vi "Process.vi"(8 "error in":errorcluster, 11 "SynchIO.USB4431":refnum<class "SynchIO.USB4431.lvclass">) -> (0 "error out":errorcluster, 3 "SynchIO.USB4431 out":refnum<class "SynchIO.USB4431.lvclass">)   [LabVIEW 2016, in "SynchIO.USB4431.lvclass"]
doc: "---------------------------------------------------------------\nJKI State Machine Objects™\nhttp://jki.net/state-machine-objects/\nCopyright (C) 2005-2015, JKI <info@jki.net>\nALL RIGHTS RESERVEDJKI State Machine Objects (SMO) 1.0.0.5\nJKI - JKI\nCopyright (c) 2016, JKI"
uses:
  SynchIO.USB4431.lvclass
  C:/Program Files (x86)/National Instruments/LabVIEW 2016/vi.lib/JKI/JKI SMO/SMO/SMO.lvclass
  <vilib>/JKI/JKI SMO/SMO/Typedefs/Parent Call--Enum.ctl
  SynchIO/SynchIO.lvclass
  <vilib>/JKI/JKI SMO/SMO/SMO.lvclass
panel:
  in  "Start":bool
  in  "stop":bool
  in  "Tab Control":T1(tab)=enum."AO Config"
  in  "AI Configuration":T2(array[cluster])=[{"AI.Coupling"=enum."DC", "AI.Max"=10.0, "AI.Min"=-10.0, "Input physical channels"="Dev1/ai0:3"}]
  in  "AO Configuration":T3(array[cluster])=[{"Output physical channels"="Dev1/ao0", "AO. Max"=3.5, "AO.Min"=-3.5}]
  in  "sampling info":cluster{"Fs":dbl, "#s":dbl}={"Fs"=102388.0, "#s"=7876.0}
  in  "AI Buffer Size (S)":i32=100
  in  "Channels: AO":T4={"AO amp (V)"=[1.0, 0.0, 0.0, 0.0, 0.0, 0.0, 0.0, 0.0], "AO DC (V)"=[0.0, 0.0, 0.0, 0.0, 0.0, 0.0, 0.0, 0.0], "AO f (Hz)"=[17.0, 13.0, 13.0, 13.0, 13.0, 13.0, 13.0, 13.0], "AO phi (deg)"=[0.0, 0.0, 0.0, 0.0, 0.0, 0.0, 0.0, 0.0], "function"=[enum."Sine Wave", enum."Sine Wave", enum."Sine Wave", enum."Sine Wave", enum."Sine Wave", enum."Sine Wave", enum."Sine Wave", enum."Sine Wave"]}
  in  "AO":T4={"AO amp (V)"=[1.0, 0.0, 0.0, 0.0, 0.0, 0.0, 0.0, 0.0], "AO DC (V)"=[0.0, 0.0, 0.0, 0.0, 0.0, 0.0, 0.0, 0.0], "AO f (Hz)"=[13.0, 13.0, 13.0, 13.0, 13.0, 13.0, 13.0, 13.0], "AO phi (deg)"=[0.0, 0.0, 0.0, 0.0, 0.0, 0.0, 0.0, 0.0], "function"=[enum."Sine Wave", enum."Sine Wave", enum."Sine Wave", enum."Sine Wave", enum."Sine Wave", enum."Sine Wave", enum."Sine Wave", enum."Sine Wave"]} {"AO DC (V)" format="%#_6p"; "AO amp (V)" format="%#_6p"}
  out "Signals Graph":waveform(dbl)[](graph)=[{"t0"=timestamp(3565974471.4961195 s since 1904-01-01), "dt"=1.0, "Y"=array[6023 elements], "attributes"=variant("NI_ChannelName"=variant(string "Dev2/ai0"), "NI_UnitDescription"=variant(string "Volts"))}, {"t0"=timestamp(3565974471.4961195 s since 1904-01-01), "dt"=1.0, "Y"=array[6023 elements], "attributes"=variant("NI_ChannelName"=variant(string "Dev2/ai1"), "NI_UnitDescription"=variant(string "Volts"))}, {"t0"=timestamp(3565974471.4961195 s since 1904-01-01), "dt"=1.0, "Y"=array[6023 elements], "attributes"=variant("NI_ChannelName"=variant(string "Dev2/ai2"), "NI_UnitDescription"=variant(string "Volts"))}, {"t0"=timestamp(3565974471.4961195 s since 1904-01-01), "dt"=1.0, "Y"=array[6023 elements], "attributes"=variant("NI_ChannelName"=variant(string "Dev2/ai3"), "NI_UnitDescription"=variant(string "Volts"))}, {"t0"=timestamp(3565974471.554943 s since 1904-01-01), "dt"=1.0, "Y"=array[6023 elements], "attributes"=variant("NI_ChannelName"=variant(string "Dev2/ai0"), "NI_UnitDescription"=variant(string "Volts"))}, {"t0"=timestamp(3565974471.554943 s since 1904-01-01), "dt"=1.0, "Y"=array[6023 elements], "attributes"=variant("NI_ChannelName"=variant(string "Dev2/ai1"), "NI_UnitDescription"=variant(string "Volts"))}]
  out "Signals Graph 2":waveform(dbl)[](graph)=[{"t0"=timestamp(3565974471.4961195 s since 1904-01-01), "dt"=1.0, "Y"=array[6023 elements], "attributes"=variant("NI_ChannelName"=variant(string "Dev2/ai0"), "NI_UnitDescription"=variant(string "Volts"))}, {"t0"=timestamp(3565974471.4961195 s since 1904-01-01), "dt"=1.0, "Y"=array[6023 elements], "attributes"=variant("NI_ChannelName"=variant(string "Dev2/ai1"), "NI_UnitDescription"=variant(string "Volts"))}, {"t0"=timestamp(3565974471.4961195 s since 1904-01-01), "dt"=1.0, "Y"=array[6023 elements], "attributes"=variant("NI_ChannelName"=variant(string "Dev2/ai2"), "NI_UnitDescription"=variant(string "Volts"))}, {"t0"=timestamp(3565974471.4961195 s since 1904-01-01), "dt"=1.0, "Y"=array[6023 elements], "attributes"=variant("NI_ChannelName"=variant(string "Dev2/ai3"), "NI_UnitDescription"=variant(string "Volts"))}, {"t0"=timestamp(3565974471.554943 s since 1904-01-01), "dt"=1.0, "Y"=array[6023 elements], "attributes"=variant("NI_ChannelName"=variant(string "Dev2/ai0"), "NI_UnitDescription"=variant(string "Volts"))}, {"t0"=timestamp(3565974471.554943 s since 1904-01-01), "dt"=1.0, "Y"=array[6023 elements], "attributes"=variant("NI_ChannelName"=variant(string "Dev2/ai1"), "NI_UnitDescription"=variant(string "Volts"))}]
  out "Current State":string="Exit"
  out "State History":string
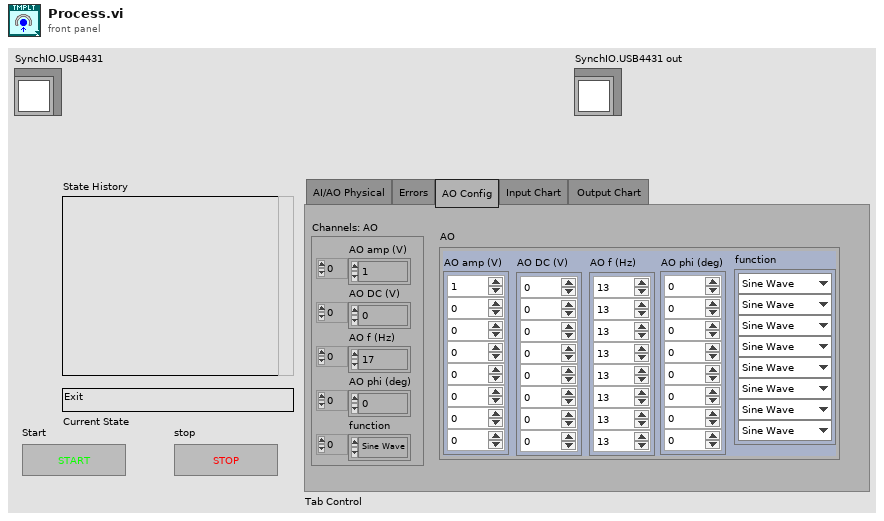
[diagram p1: front panel]
types:
  T1 = enum32{"AI/AO Physical", "Errors", "AO Config", "Input Chart", "Output Chart "}
  T2 = cluster{"AI.Coupling":enum16{"AC", "DC", "GND"}, "AI.Max":dbl, "AI.Min":dbl, "Input physical channels":tag}[]
  T3 = cluster{"Output physical channels":tag, "AO. Max":dbl, "AO.Min":dbl}[]
  T4 = cluster{"AO amp (V)":dbl[], "AO DC (V)":dbl[], "AO f (Hz)":dbl[], "AO phi (deg)":dbl[], "function":enum16{"Sine Wave", "Triangle Wave", "Square Wave", "Sawtooth Wave"}[]}
  T5 = typedef "SMO.lvclass/Parent Call--Enum.ctl" = enum16{"Allows parent to run", "Does not request parent to run"}
  T6 = enum32{"invalid app kind", "Development System", "Run Time System", "Student Edition", "Embedded LabVIEW", "Evaluation", "Custom"}
  T7 = enum32{"Invalid", "Standard", "Closed", "Hidden", "Minimized", "Maximized"}
  T8 = cluster{"Core":cluster{"Current VI Reference":refnum<vi>, "Close Panel on Exit?":bool, "error":errorcluster}, "Self Reference":refnum<class "SynchIO.USB4431.lvclass">, "Your string data":string, "AI Buffer Size (S)":i32, "AI Configuration":cluster{"AI.Coupling":enum16{"AC", "DC", "GND"}, "AI.Max":dbl, "AI.Min":dbl, "Input physical channels":tag}[], "AO Configuration":cluster{"Output physical channels":tag, "AO. Max":dbl, "AO.Min":dbl}[], "Channels: AO":cluster{"AO amp (V)":dbl[], "AO DC (V)":dbl[], "AO f (Hz)":dbl[], "AO phi (deg)":dbl[], "function":enum16{"Sine Wave", "Triangle Wave", "Square Wave", "Sawtooth Wave"}[]}, "sampling info":cluster{"Fs":dbl, "#s":dbl}, "AI task":refnum<k21>[], "AO Task":refnum<k21>[], "AI Data":waveform(dbl)[], "AO Data":waveform(dbl)[], "AO":cluster{"AO amp (V)":dbl[], "AO DC (V)":dbl[], "AO f (Hz)":dbl[], "AO phi (deg)":dbl[], "function":enum16{"Sine Wave", "Triangle Wave", "Square Wave", "Sawtooth Wave"}[]}, "Iteration":i32}
  T9 = cluster{"Current VI Reference":refnum<vi>, "Close Panel on Exit?":bool, "error":errorcluster}
  T10 = typedef "SMO.lvclass/Protected Events.ctl" = cluster{"StopProcesses":refnum<user-event>, "AbortProcesses":refnum<user-event>, "Config Changed":refnum<user-event>, "Dependency":refnum<user-event>}
  T11 = typedef "SynchIO.USB4431.lvclass/ProtectedEvents--Cluster.ctl" = cluster{"API_Template":refnum<user-event>}
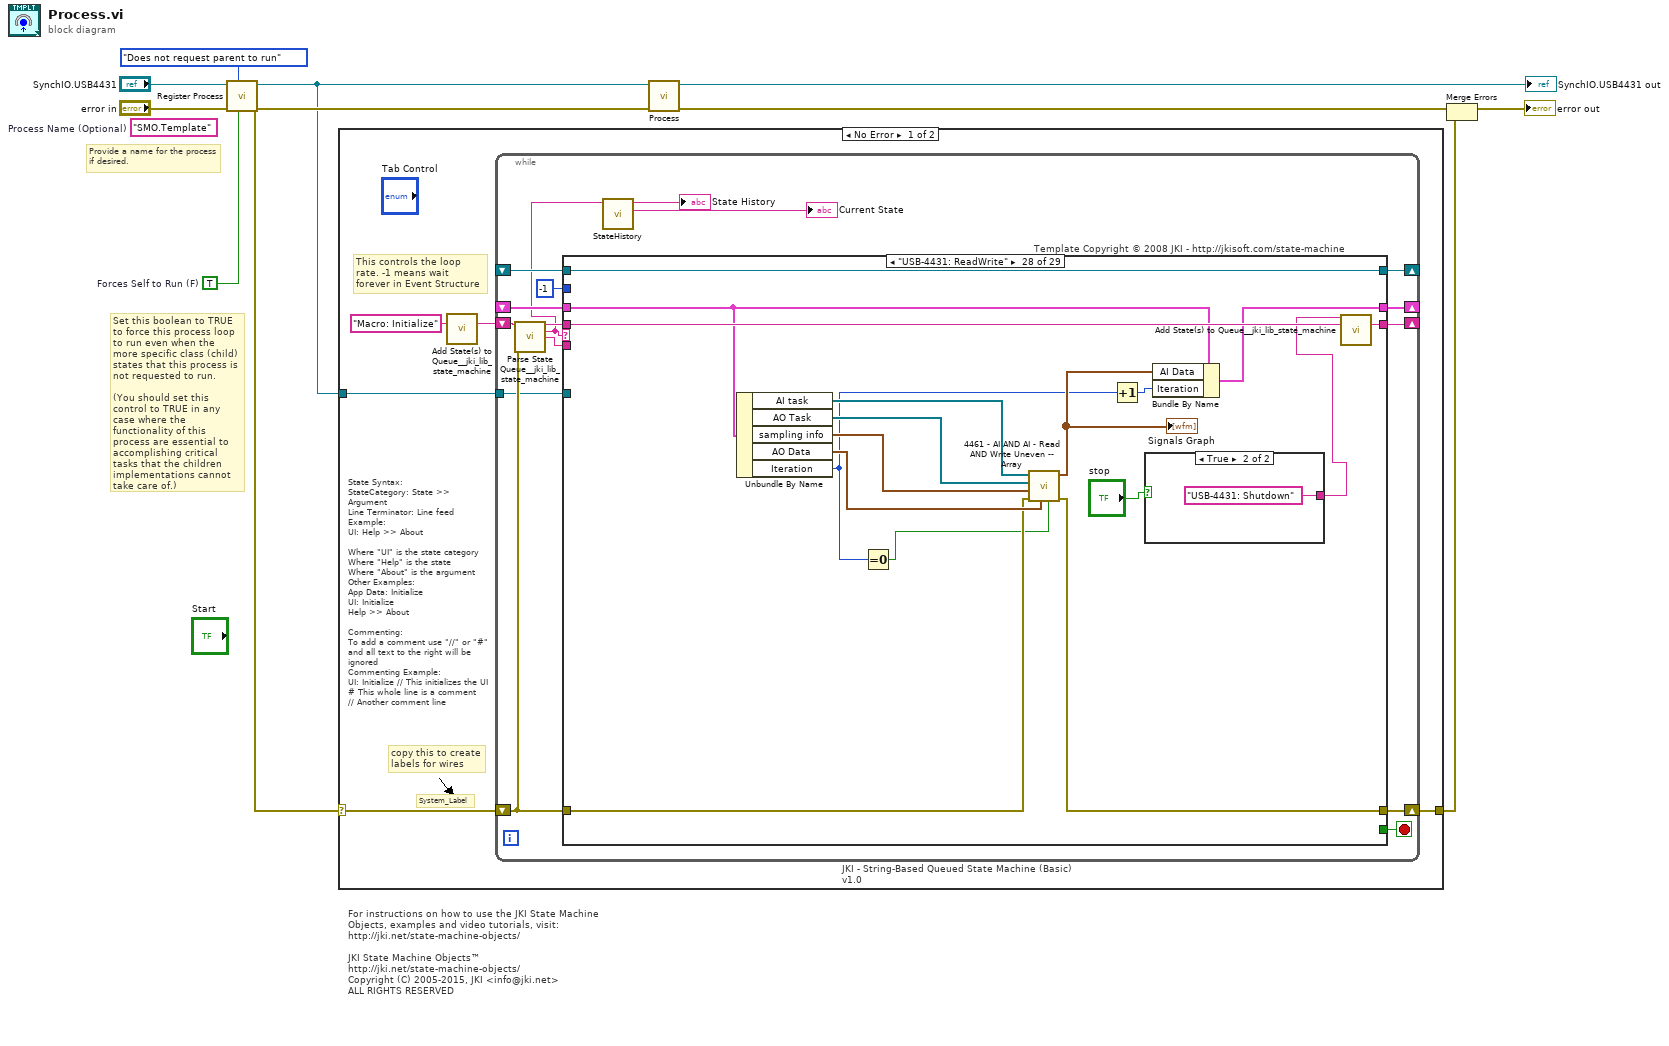
[diagram p0: block diagram]
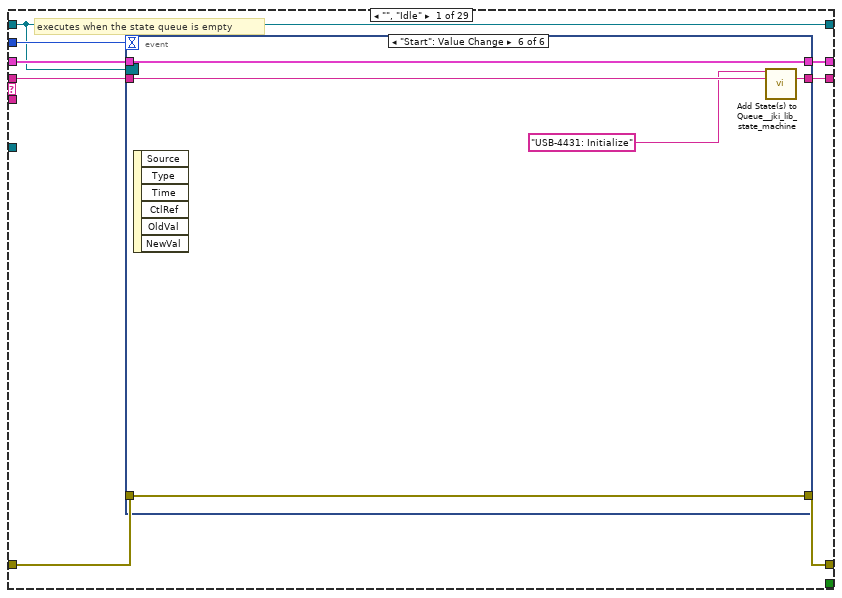
[diagram p2: hidden frame]
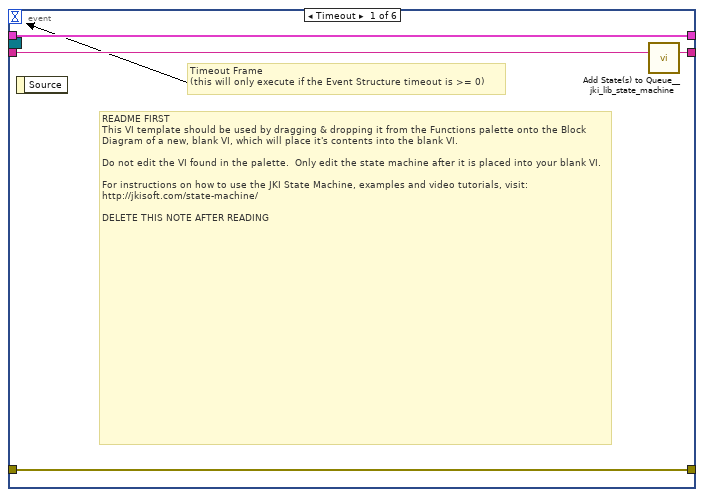
[diagram p3: hidden frame]
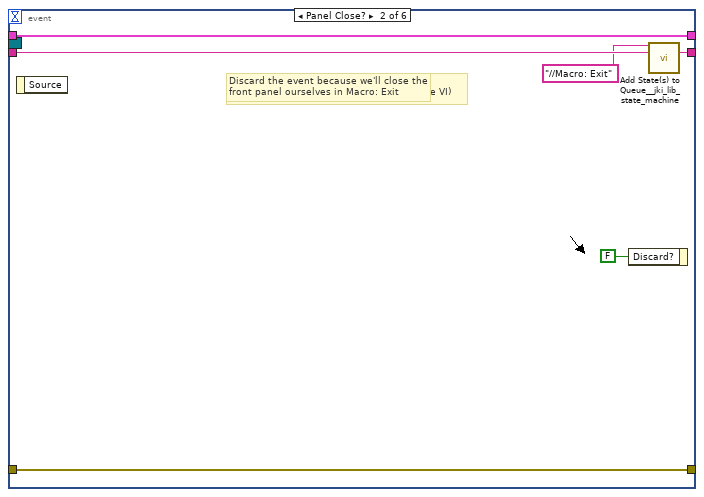
[diagram p4: hidden frame]
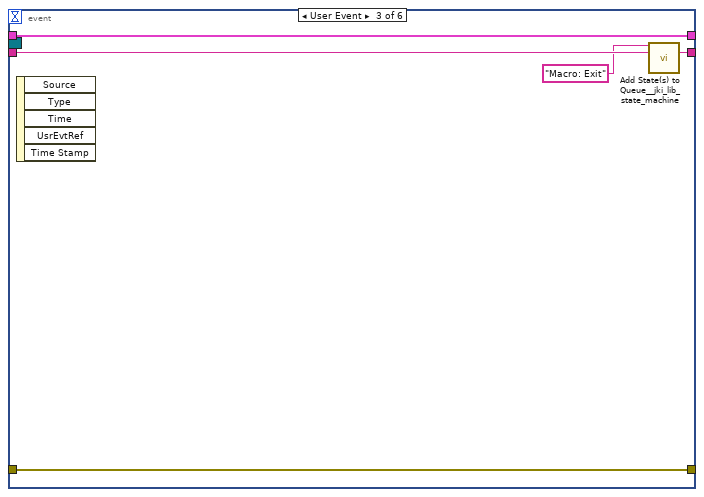
[diagram p5: hidden frame]
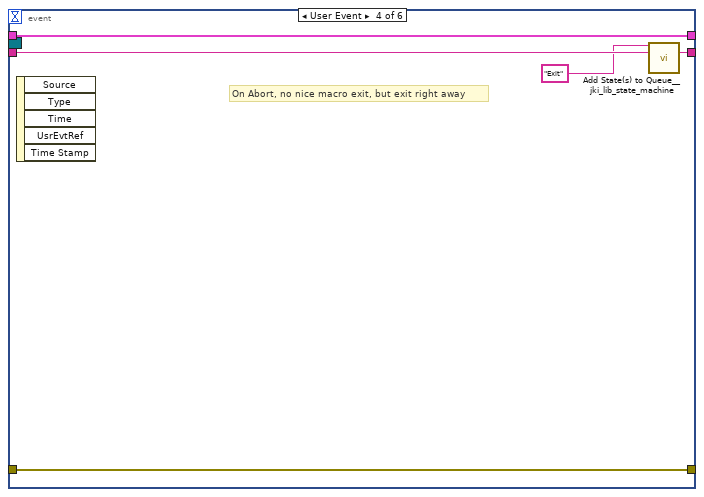
[diagram p6: hidden frame]
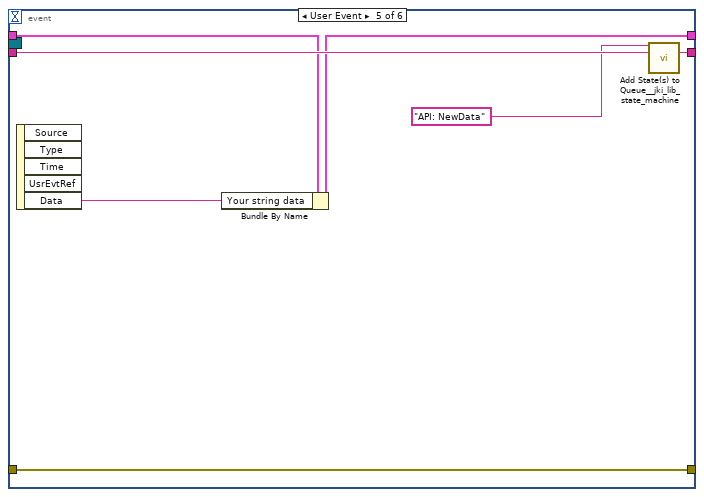
[diagram p7: hidden frame]
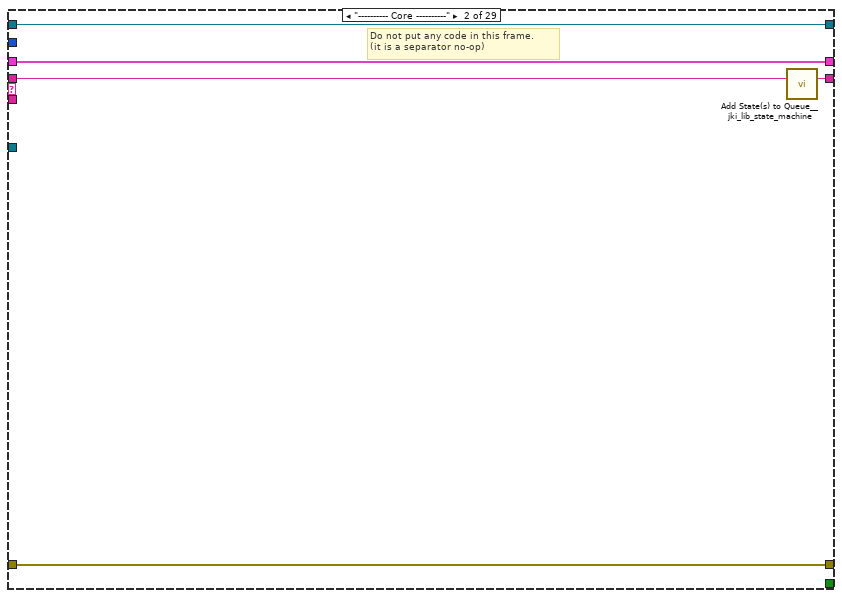
[diagram p8: hidden frame]
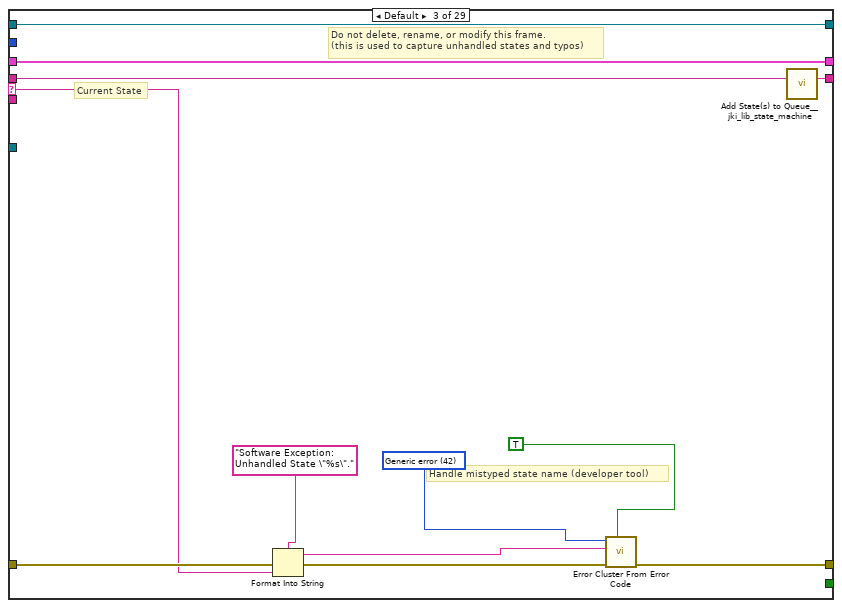
[diagram p9: hidden frame]
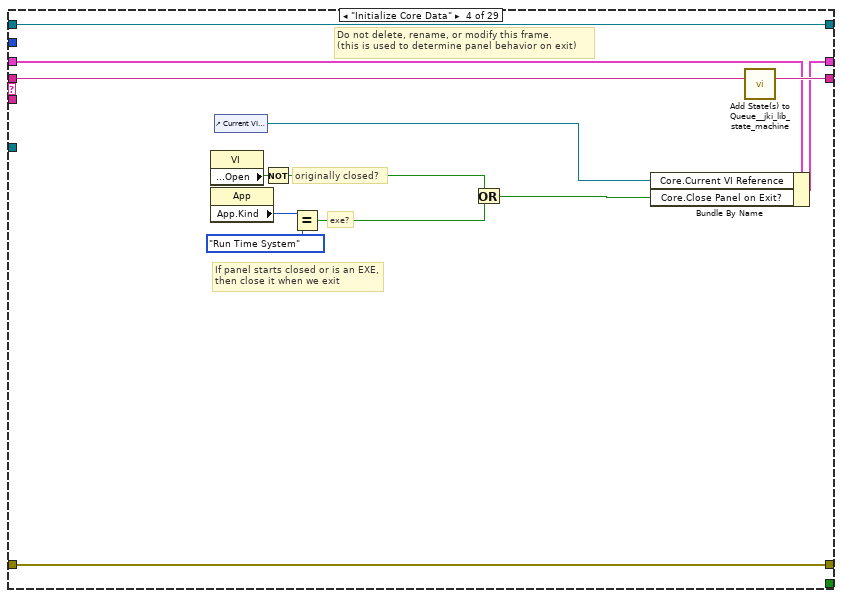
[diagram p10: hidden frame]
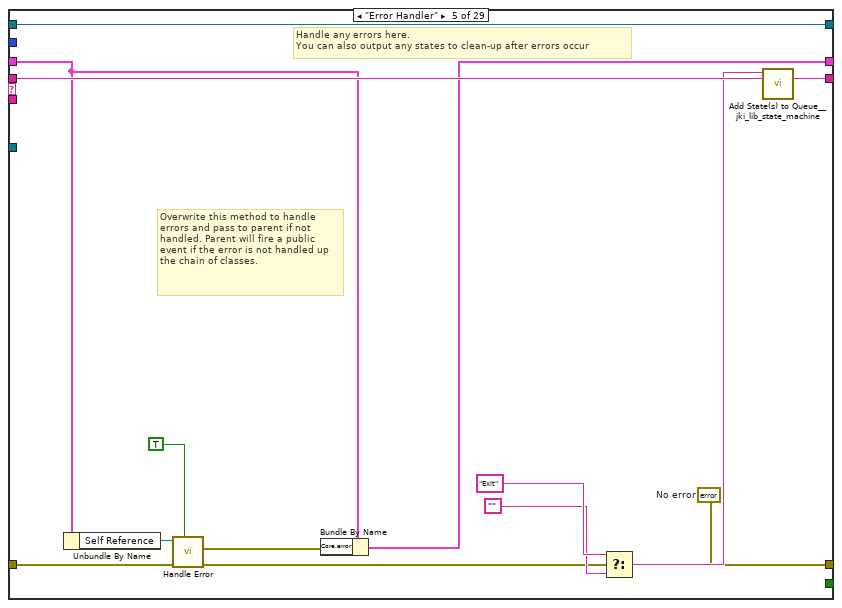
[diagram p11: hidden frame]
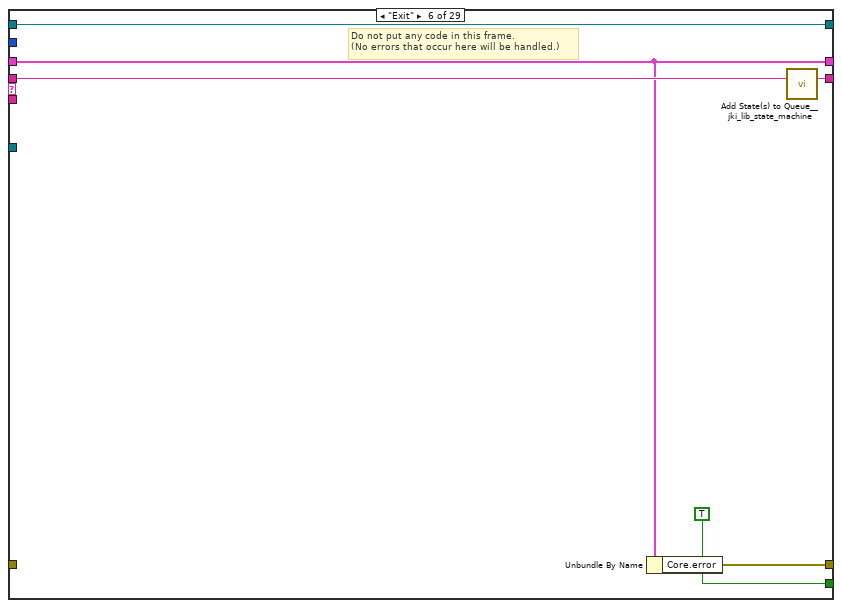
[diagram p12: hidden frame]
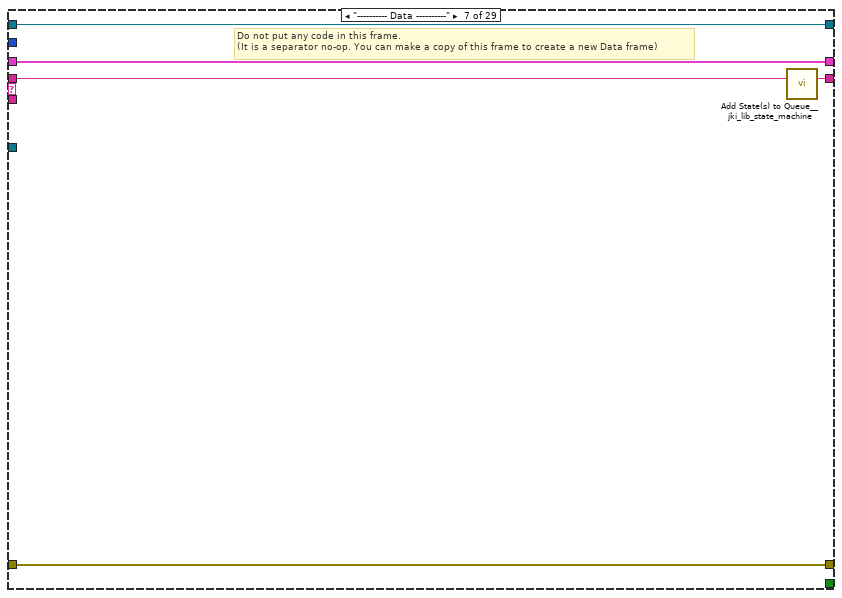
[diagram p13: hidden frame]
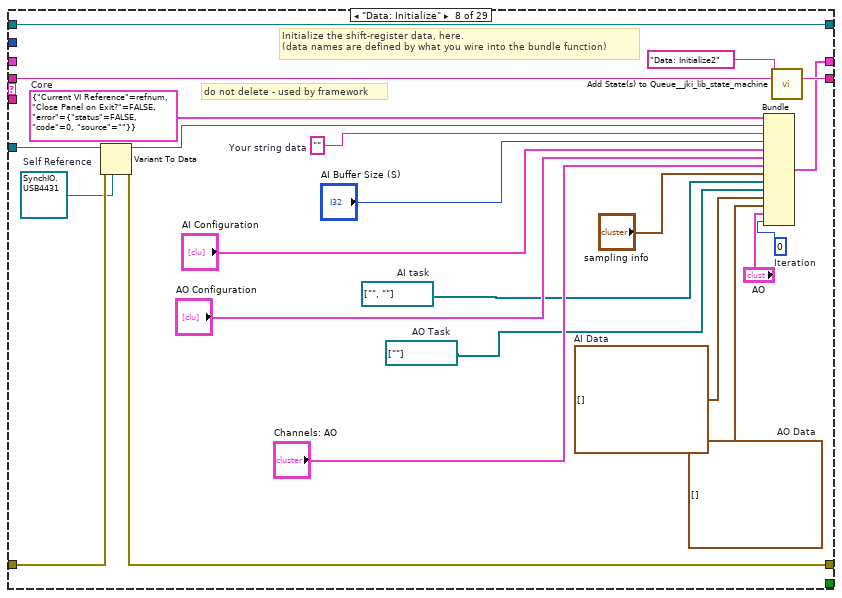
[diagram p14: hidden frame]
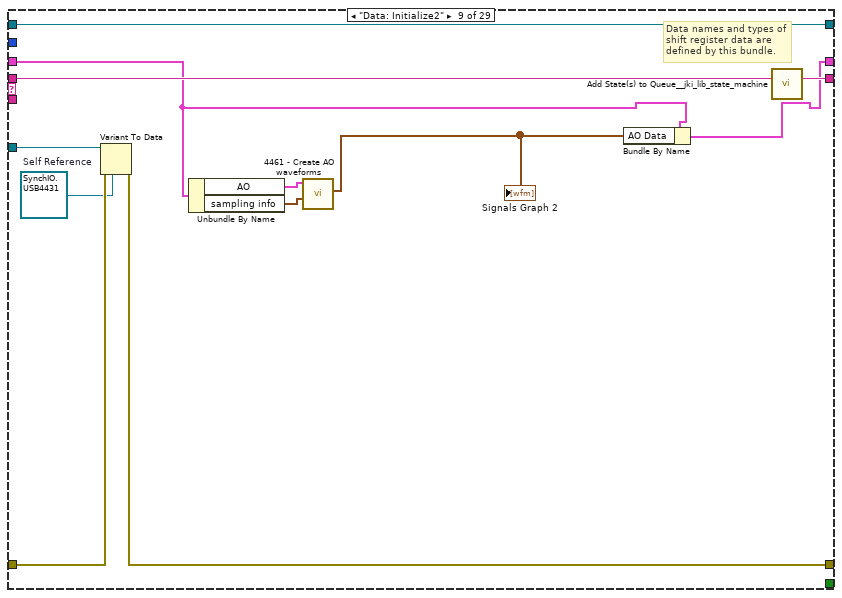
[diagram p15: hidden frame]
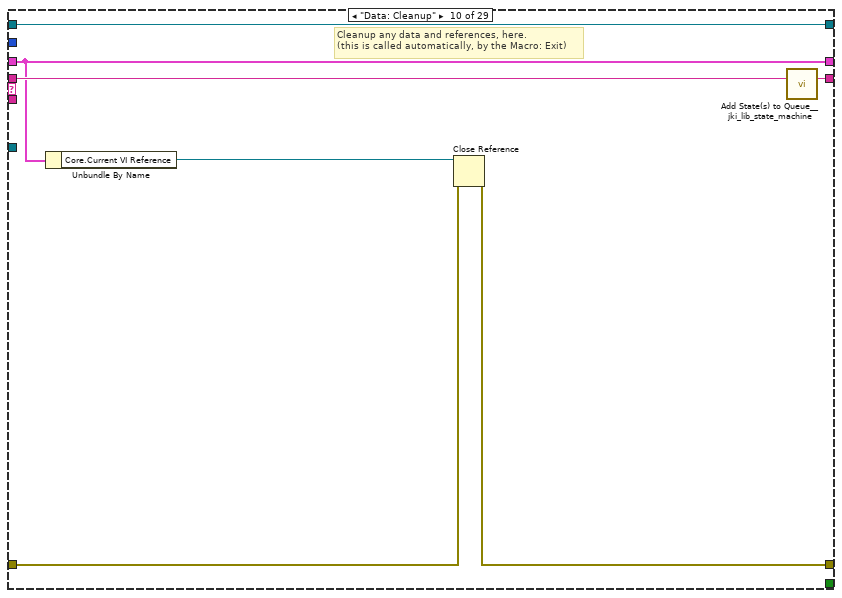
[diagram p16: hidden frame]
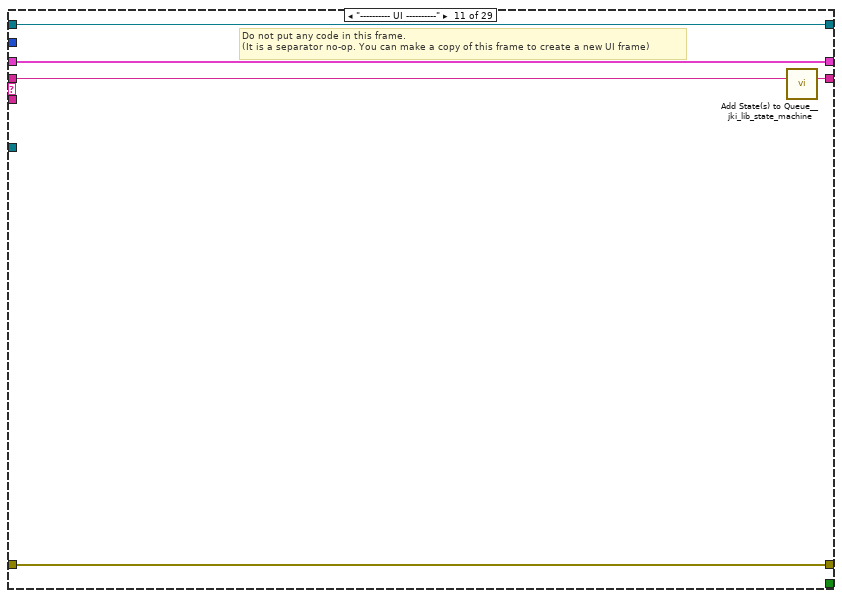
[diagram p17: hidden frame]
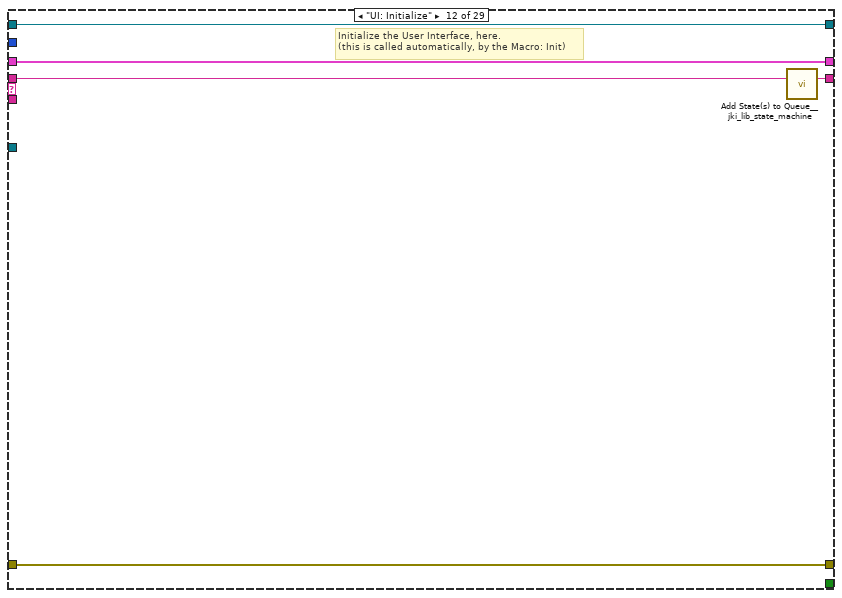
[diagram p18: hidden frame]
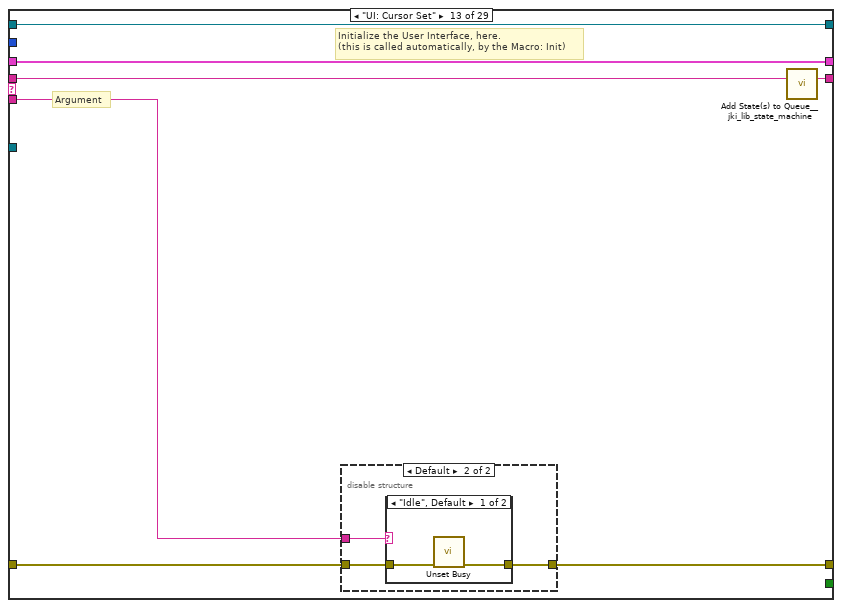
[diagram p19: hidden frame]
diagram:
  w1 = TRUE  # Forces Self to Run (F)
  (unwired) "SMO.Template"  # Process Name (Optional)
  # "Provide a name for the process\nif desired."
  # "Set this boolean to TRUE to force this process loop to run even when the more specific class (child) states that this process is not requested to run.\n\n(You should set this control to TRUE in any case where the functionality of this process are essential to accomplishing critical tasks that the children implementations cannot take care of.)"
  # "For instructions on how to use the JKI State Machine Objects, examples and video tutorials, visit:\nhttp://jki.net/state-machine-objects/\n\nJKI State Machine Objects™\nhttp://jki.net/state-machine-objects/\nCopyright (C) 2005-2015, JKI <info@jki.net>\nALL RIGHTS RESERVED"
  n1 = call <vilib>:"Register Process.vi"("Forces Self to Run (F)"=w1, "Parent Call"=Parent_Call--Enum."Does not request parent to run", "error in (no error)"="error in", "SMO"="SynchIO.USB4431") -> ("error out"=w7:errorcluster, "SMO out"=w6:refnum<class "SynchIO.USB4431.lvclass">)  [unwired: 6 in]
  n2 = case shown="No Error" w7 {
    selector: w7 -> [w12 w378]
    tunnel: w6 -> [w13 _]
    tunnel: [w11 w378] -> w3
    frame No Error {
      # "State Syntax:\nStateCategory: State >> Argument\nLine Terminator: Line feed\nExample:\nUI: Help >> About\n\nWhere \"UI\" is the state category\nWhere \"Help\" is the state\nWhere \"About\" is the argument\nOther Examples:\nApp Data: Initialize\nUI: Initialize\nHelp >> About\n\nCommenting:\nTo add a comment use \"//\" or \"#\" and all text to the right will be ignored\nCommenting Example:\nUI: Initialize // This initializes the UI\n# This whole line is a comment\n// Another comment line"
      # "copy this to create labels for wires"
      # "This controls the loop rate. -1 means wait forever in Event Structure"
      # "System_Label"
      n3 = call <vilib>:"Add State(s) to Queue__jki_lib_state_machine.vi"("State(s) in (\"\")"="Macro: Initialize") -> ("States Out"=w15:string)  [unwired: 14 in]
      n4 = while "JKI - String-Based Queued State Machine (Basic) v1.0" {
        shift-right: [w26] -> _
        shift-left: _ -> [w25]
        shift-right: [w29] -> w11
        shift-left: w12 -> [w23]
        shift-right: [w28] -> _
        shift-left: w15 -> [w30]
        tunnel: w13 -> [w22]
        shift-right: [w21] -> _
        shift-left: _ -> [w20]
        stop <- w27 stop-if-true
        # "Template Copyright © 2008 JKI - http://jkisoft.com/state-machine"
        n5 = call <vilib>:"Parse State Queue__jki_lib_state_machine.vi"("State Queue"=w30, "Error In (no error)"=w23) -> ("Remaining States"=w17:string, "Current State"=w16:string, "Arguments"=w31:string)  [unwired: 11 in]
        n6 = case shown="\"USB-4431: ReadWrite\"" w16 {
          selector: w16 -> [_ _ w78 _ _ _ _ _ _ _ _ _ _ _ _ _ _ _ _ _ _ _ _ _ _ _ _ _ _]
          tunnel: w17 -> [w39 w76 w82 w101 w115 w121 w126 w149 w161 w168 w173 w178 w185 w201 w233 w242 w256 w261 w272 w277 w290 w296 w301 w309 w314 w319 w335 w352 w364]
          tunnel: w31 -> [_ _ _ _ _ _ _ _ _ _ _ _ w179 w195 _ _ _ _ _ _ _ _ _ _ _ _ _ _ _]
          tunnel: w25 -> [w37 w73 w80 w92 w104 w117 w123 _ w152 w163 w170 w176 w183 w197 w230 w238 w247 w258 w269 w274 w288 w294 w299 w306 w311 w317 w328 w349 w359]
          tunnel: [w36 w74 w84 w98 w106 w116 w124 w144 w158 w164 w171 w175 w180 w198 w231 w240 w254 w259 w263 w275 w278 w292 w297 w303 w310 w315 w324 w344 w361] -> w29
          tunnel: w23 -> [w35 w74 w83 w98 w111 _ w124 w145 w159 w165 w171 w175 w181 w199 w231 w240 w254 w259 w264 w275 w282 w292 w297 w304 w310 w315 w325 w339 w360]
          tunnel: [w38 w75 w81 w100 w114 w120 w125 w148 w160 w167 w172 w177 w184 w200 w232 w241 w255 w260 w271 w276 w289 w295 w300 w308 w313 w318 w334 w351 w363] -> w28
          tunnel: [_ _ _ _ _ TRUE _ _ _ _ _ _ _ _ _ _ _ _ _ _ _ _ _ _ _ _ _ _ _] -> w27
          tunnel: [w34 w73 w80 w99 w103 w117 w123 w147 w151 w163 w170 w176 w183 w197 w230 w238 w247 w258 w269 w274 w288 w294 w299 w306 w311 w317 w327 w348 w359] -> w26
          tunnel: -1 ("Timeout") -> [w33 _ _ _ _ _ _ _ _ _ _ _ _ _ _ _ _ _ _ _ _ _ _ _ _ _ _ _ _]
          tunnel: w22 -> [_ _ _ _ _ _ _ w142 w156 _ _ _ _ _ _ _ _ _ _ _ _ _ _ _ _ _ _ _ _]
          tunnel: [w32 w72 w77 w89 w113 w118 w122 w140 w155 w162 w169 w174 w182 w194 w229 w239 w248 w257 w270 w273 w287 w293 w298 w307 w312 w316 w333 w350 w362] -> w21
          tunnel: w20 -> [w32 w72 w77 w89 w113 w118 w122 w140 w155 w162 w169 w174 w182 w194 w229 w239 w248 w257 w270 w273 _ w293 w298 w307 w312 w316 w333 w350 w362]
          frame "", "Idle" {
            # "executes when the state queue is empty"
            n7 = event shown="[5] \"Start\": Value Change" {
              selector: w32 -> [_ _ _ _ _ _]
              dyn-events: _ -> [_ _ _ _ _ _]
              timeout: w33 -> [_ _ _ _ _ _]
              tunnel: w39 -> [w43 w49 w54 w59 w66 w71]
              tunnel: [w42 w48 w53 w58 w65 w70] -> w38
              tunnel: w37 -> [w40 w46 w51 w56 w63 w67]
              tunnel: [w41 w47 w52 w57 w64 w69] -> w36
              tunnel: w35 -> [w41 w47 w52 w57 w64 w69]
              tunnel: [w40 w46 w51 w56 w62 w67] -> w34
              event Timeout {
                # "README FIRST\nThis VI template should be used by dragging & dropping it from the Functions palette onto the Block Diagram of a new, blank VI, which will place it's contents into the blank VI.\n\nDo not edit the VI found in the palette.  Only edit the state machine after it is placed into your blank VI.\n\nFor instructions on how to use the JKI State Machine, examples and video tutorials, visit:\nhttp://jkisoft.com/state-machine/\n\nDELETE THIS NOTE AFTER READING"
                # "Timeout Frame\n(this will only execute if the Event Structure timeout is >= 0)"
                n8 = event-data() -> ()  [unwired: 1 in, 1 out]
                n9 = call <vilib>:"Add State(s) to Queue__jki_lib_state_machine.vi"("State(s) in (\"\")"=w43) -> ("States Out"=w42:string)  [unwired: 14 in]
              }
              event Panel Close? {
                # "Discard the event because we'll close the front panel ourselves in Macro: Exit"
                # "Close Panel button (pressed) Event\n(this executes Macro: Exit to terminate the VI)"
                n10 = event-data() -> ()  [unwired: 1 in, 1 out]
                n11 = event-data("Discard?"=FALSE) -> ()  [unwired: 1 in, 1 out]
                n12 = call <vilib>:"Add State(s) to Queue__jki_lib_state_machine.vi"("State(s) in Front (\"\")"="//Macro: Exit", "State(s) in (\"\")"=w49) -> ("States Out"=w48:string)  [unwired: 13 in]
              }
              event User Event {
                n13 = event-data() -> ()  [unwired: 1 in, 5 out]
                n14 = call <vilib>:"Add State(s) to Queue__jki_lib_state_machine.vi"("State(s) in Front (\"\")"="Macro: Exit", "State(s) in (\"\")"=w54) -> ("States Out"=w53:string)  [unwired: 13 in]
              }
              event User Event {
                # "On Abort, no nice macro exit, but exit right away"
                n15 = event-data() -> ()  [unwired: 1 in, 5 out]
                n16 = call <vilib>:"Add State(s) to Queue__jki_lib_state_machine.vi"("State(s) in Front (\"\")"="Exit", "State(s) in (\"\")"=w59) -> ("States Out"=w58:string)  [unwired: 13 in]
              }
              event User Event {
                n17 = event-data() -> ("Data"=w60:string)  [unwired: 1 in, 4 out]
                n18 = Bundle By Name(cluster=w63, "Your string data"=w60) -> (w62:T8)
                n19 = call <vilib>:"Add State(s) to Queue__jki_lib_state_machine.vi"("State(s) in Front (\"\")"="API: NewData", "State(s) in (\"\")"=w66) -> ("States Out"=w65:string)  [unwired: 13 in]
              }
              event "Start": Value Change {
                n20 = event-data() -> ()  [unwired: 1 in, 6 out]
                n21 = call <vilib>:"Add State(s) to Queue__jki_lib_state_machine.vi"("State(s) in Front (\"\")"="USB-4431: Initialize", "State(s) in (\"\")"=w71) -> ("States Out"=w70:string)  [unwired: 13 in]
              }
            }
          }
          frame "---------- Core ----------" {
            # "Do not put any code in this frame.\n(it is a separator no-op)"
            n22 = call <vilib>:"Add State(s) to Queue__jki_lib_state_machine.vi"("State(s) in (\"\")"=w76) -> ("States Out"=w75:string)  [unwired: 14 in]
          }
          frame Default {
            w87 = 42 items=["No error", "Argument error", "Memory is full", "Out of zone", "End of file", "File already open", "Generic file I/O error", "File not found", "File permission error", "Disk is full", "Duplicate path", "Too many files open", "System feature not enabled", "Resource file not found", "Cannot add resource", "Resource not found", "Image not found", "Image memory error", "Pen does not exist", "Config type invalid", "Config token not found", "Config parse error", "Config memory error", "Bad external code format", "Bad external code offset", "External code not present", "Null window", "Destroy window error", "Null menu", "Print aborted", "Bad print record", "Print driver error", "Windows error during printing", "Memory error during printing", "Print dialog error", "Generic print error", "Invalid device refnum", "Device not found", "Device parameter error", "Device unit error", "Cannot open device", "Device call aborted", "Generic error", "Cancelled by user", "Object ID too low", "Object ID too high", "Object not in heap", "Unknown heap", "Unknown object (invalid DefProc)", "Unknown object (DefProc not in table)", "Message out of range", "Invalid (null) method", "Unknown message", "Manager call not supported", "Bad address", "Network operation in progress", "Network operation timed out", "Connection is busy", "Network attribute not supported", "Network error", "Address in use", "System out of memory", "Connection aborted", "Connection refused", "Not connected", "Already connected", "Connection closed", "Initialization error (interapplication manager)", "Bad occurrence", "Wait on unbound occurrence handler", "Occurrence queue overflow", "Datalog type conflict", "Unused", "Unrecognized type (interapplication manager)", "Memory corrupt", "Failed to make temporary DLL", "Old CIN version", "Drag socket not found", "Failed to load drop-object", "Failed to register OLE object", "Failed to release OLE object", "Format specifier type mismatch", "Unknown format specifier", "Too few format specifiers", "Too many format specifiers", "Scan failed", "Newer CIN version", "Error converting to variant", "Runtime menu error", "Password tampered", "Variant attribute not found", "Incompatible variant data type", "Event data is not available", "Event Store is not present", "Occurrence is not found", "Event Queue is not created", "Event info is not available", "Refnum passed is NULL", "Error retrieving Class GUID", "Error retrieving CoClass GUID", "Error retrieving TypeLib GUID.", "Bad built application magic bytes.", "Specific driver is different from the specific driver associated with the Logical Name.", "There is no session opened to the class driver.", "Max Error", "MAX - Error with config objects", "MAX - Error loading configuration", "MAX - Group not supported"]
            # "Current State"
            # "Do not delete, rename, or modify this frame.\n(this is used to capture unhandled states and typos)"
            # "Handle mistyped state name (developer tool)"
            n23 = Format Into String(format string="Software Exception: Unhandled State \"%s\"." ("message"), error in=w83, w78) -> (resulting string=w86:string, error out=w85:errorcluster)  [unwired: 1 in]
            n24 = call <vilib>:"Error Cluster From Error Code.vi"("show call chain? (False)"=TRUE, "error in (no error)"=w85, "error message (\"\")"=w86, "error code (0)"=w87) -> ("error out"=w84:errorcluster)  [unwired: 5 in]
            n25 = call <vilib>:"Add State(s) to Queue__jki_lib_state_machine.vi"("State(s) in (\"\")"=w82) -> ("States Out"=w81:string)  [unwired: 14 in]
          }
          frame "Initialize Core Data" {
            # "Do not delete, rename, or modify this frame.\n(this is used to determine panel behavior on exit)"
            # "originally closed?"
            # "exe?"
            # "If panel starts closed or is an EXE, then close it when we exit"
            n26 = property class="VI"() -> ("Front Panel.Open"=w97:bool)  [unwired: 2 in, 2 out]
            n27 = property class="App"() -> ("App.Kind"=w96:T6)  [unwired: 2 in, 2 out]
            n28 = control-ref of="Current VI Reference"() -> (w90:refnum<vi>)
            n29 = Not(x=w97) -> (.not. x?=w94:bool)
            n30 = Equal?(x=w96, y=T6."Run Time System" ("Application:Kind")) -> (x = y?=w93:bool)
            n31 = Or(x=w94, y=w93) -> (x .or. y?=w91:bool)
            n32 = Bundle By Name(cluster=w92, "Core.Current VI Reference"=w90, "Core.Close Panel on Exit?"=w91) -> (w99:T8)
            n33 = call <vilib>:"Add State(s) to Queue__jki_lib_state_machine.vi"("State(s) in (\"\")"=w101) -> ("States Out"=w100:string)  [unwired: 14 in]
          }
          frame "Error Handler" {
            w106 = errorcluster {"status"=FALSE, "code"=0, "source"=""}  # No error
            # "Overwrite this method to handle errors and pass to parent if not handled. Parent will fire a public event if the error is not handled up the chain of classes."
            # "Handle any errors here.\nYou can also output any states to clean-up after errors occur"
            n34 = Unbundle By Name(w104) -> ("Self Reference"=w112:refnum<class "SynchIO.USB4431.lvclass">)
            n35 = call-dynamic "Handle Error.vi"("Stop on Unhandled Error (T)"=TRUE, "error in"=w111, "SMO"=w112) -> ("handling error"=w107:errorcluster, "Unhandled error"=w105:errorcluster)  [unwired: 6 in, 1 out]
            n36 = Bundle By Name(cluster=w104, "Core.error"=w105) -> (w103:T8)
            n37 = Select(t="Exit", s=w107, f="") -> (s? t:f=w108:string)
            n38 = call <vilib>:"Add State(s) to Queue__jki_lib_state_machine.vi"("State(s) in Front (\"\")"=w108, "State(s) in (\"\")"=w115) -> ("States Out"=w114:string)  [unwired: 13 in]
          }
          frame "Exit" {
            # "Do not put any code in this frame.\n(No errors that occur here will be handled.)"
            n39 = Unbundle By Name(w117) -> ("Core.error"=w116:errorcluster)
            n40 = call <vilib>:"Add State(s) to Queue__jki_lib_state_machine.vi"("State(s) in (\"\")"=w121) -> ("States Out"=w120:string)  [unwired: 14 in]
          }
          frame "---------- Data ----------" {
            # "Do not put any code in this frame.\n(It is a separator no-op. You can make a copy of this frame to create a new Data frame)"
            n41 = call <vilib>:"Add State(s) to Queue__jki_lib_state_machine.vi"("State(s) in (\"\")"=w126) -> ("States Out"=w125:string)  [unwired: 14 in]
          }
          frame "Data: Initialize" {
            w127 = 0  # Iteration
            w129 = waveform(dbl)[] []  # AO Data
            w130 = refnum<k21>[] [""]  # AO Task
            w131 = refnum<k21>[] ["", ""]  # AI task
            w135 = waveform(dbl)[] []  # AI Data
            w139 = T9 {"Current VI Reference"=refnum, "Close Panel on Exit?"=FALSE, "error"={"status"=FALSE, "code"=0, "source"=""}}  # Core
            w143 = refnum<class "SynchIO.USB4431.lvclass"> refnum  # Self Reference
            w146 = ""  # Your string data
            # "do not delete - used by framework"
            # "Initialize the shift-register data, here.\n(data names are defined by what you wire into the bundle function)"
            n42 = Variant To Data(error in=w145, type=w143, Variant=w142) -> (data=w141:refnum<class "SynchIO.USB4431.lvclass">, error out=w144:errorcluster)
            n43 = Bundle("Core"=w139, "Self Reference"=w141, "Your string data"=w146, "AI Buffer Size (S)"="AI Buffer Size (S)", "AI Configuration"="AI Configuration", "AO Configuration"="AO Configuration", "Channels: AO"="Channels: AO", "sampling info"="sampling info", "AI task"=w131, "AO Task"=w130, "AI Data"=w135, "AO Data"=w129, "AO"="AO", "Iteration"=w127) -> (w147:T8)  [unwired: 1 in]
            n44 = call <vilib>:"Add State(s) to Queue__jki_lib_state_machine.vi"("State(s) in Front (\"\")"="Data: Initialize2" ("State(s) in Front (\"\")"), "State(s) in (\"\")"=w149) -> ("States Out"=w148:string)  [unwired: 13 in]
          }
          frame "Data: Initialize2" {
            w157 = refnum<class "SynchIO.USB4431.lvclass"> refnum  # Self Reference
            # "Data names and types of shift register data are defined by this bundle."
            n45 = Variant To Data(error in=w159, type=w157, Variant=w156) -> (error out=w158:errorcluster)  [unwired: 1 out]
            n46 = Unbundle By Name(w152) -> ("AO"=w153:T4, "sampling info"=w154:cluster{"Fs":dbl, "#s":dbl})
            n47 = call "4461 - Create AO waveforms.vi"("sampling info"=w154, "AO"=w153) -> ("AO Array"=w150:waveform(dbl)[])  [unwired: 6 in, 3 out]
            "Signals Graph 2" <- w150
            n48 = Bundle By Name(cluster=w152, "AO Data"=w150) -> (w151:T8)
            n49 = call <vilib>:"Add State(s) to Queue__jki_lib_state_machine.vi"("State(s) in (\"\")"=w161) -> ("States Out"=w160:string)  [unwired: 14 in]
          }
          frame "Data: Cleanup" {
            # "Cleanup any data and references, here.\n(this is called automatically, by the Macro: Exit)"
            n50 = Unbundle By Name(w163) -> ("Core.Current VI Reference"=w166:refnum<vi>)
            n51 = Close Reference(reference=w166, error in (no error)=w165) -> (error out=w164:errorcluster)
            n52 = call <vilib>:"Add State(s) to Queue__jki_lib_state_machine.vi"("State(s) in (\"\")"=w168) -> ("States Out"=w167:string)  [unwired: 14 in]
          }
          frame "---------- UI ----------" {
            # "Do not put any code in this frame.\n(It is a separator no-op. You can make a copy of this frame to create a new UI frame)"
            n53 = call <vilib>:"Add State(s) to Queue__jki_lib_state_machine.vi"("State(s) in (\"\")"=w173) -> ("States Out"=w172:string)  [unwired: 14 in]
          }
          frame "UI: Initialize" {
            # "Initialize the User Interface, here.\n(this is called automatically, by the Macro: Init)"
            n54 = call <vilib>:"Add State(s) to Queue__jki_lib_state_machine.vi"("State(s) in (\"\")"=w178) -> ("States Out"=w177:string)  [unwired: 14 in]
          }
          frame "UI: Cursor Set" {
            # "Argument"
            # "Initialize the User Interface, here.\n(this is called automatically, by the Macro: Init)"
            n55 = disable-structure shown="Default" {
              disable-tunnel: w181 -> [w186 w189]
              disable-tunnel: [w186 w188] -> w180
              disable-tunnel: w179 -> [_ w187]
              frame condition #0 {
              }
              frame condition #1 (active) {
                n56 = case shown="\"Idle\", Default" w187 {
                  tunnel: w189 -> [w191 w193]
                  tunnel: [w190 w192] -> w188
                  frame "Idle", Default {
                    n57 = call <vilib>:"Unset Busy.vi"("error in (no error)"=w191) -> ("error out"=w190:errorcluster)  [unwired: 10 in]
                  }
                  frame "Busy" {
                    n58 = call <vilib>:"Set Busy.vi"("error in (no error)"=w193) -> ("error out"=w192:errorcluster)  [unwired: 9 in, 1 out]
                  }
                }
              }
            }
            n59 = call <vilib>:"Add State(s) to Queue__jki_lib_state_machine.vi"("State(s) in (\"\")"=w185) -> ("States Out"=w184:string)  [unwired: 14 in]
          }
          frame "UI: Front Panel State" {
            # "Argument"
            # "Set Front Panel Open or Closed\n(Usage: \"UI: Front Panel State >> Open|Close\")"
            n60 = Unbundle By Name(w197) -> ("Core.Current VI Reference"=w196:refnum<vi>)
            n61 = disable-structure shown="Default" {
              disable-tunnel: w199 -> [w205 w228]
              disable-tunnel: [w204 w228] -> w198
              disable-tunnel: w196 -> [w203 _]
              disable-tunnel: w195 -> [w202 _]
              frame condition #0 (active) {
                n62 = case shown="\"Open\", Default" w202 {
                  tunnel: w205 -> [w209 w222]
                  tunnel: [w211 w223] -> w204
                  tunnel: w203 -> [w210 w220]
                  frame "Open", Default {
                    n63 = property class="VI"(reference=w210, error in=w209) -> (reference out=w207:refnum<vi>, error out=w208:errorcluster, "FP.State"=w206:T7)
                    n64 = case shown="\"Closed\"" w206 {
                      tunnel: [w214 w217] -> w211
                      tunnel: w208 -> [w213 w217]
                      tunnel: w207 -> [w212 _]
                      frame "Closed" {
                        n65 = invoke class="VI" method="FP.Open"(reference=w212, error in=w213, "Activate"=TRUE, "State"=T7."Standard") -> (error out=w214:errorcluster)  [unwired: 1 in, 4 out]
                      }
                      frame Default {
                      }
                    }
                  }
                  frame "Close" {
                    n66 = property class="VI"(reference=w220, error in=w222) -> (reference out=w219:refnum<vi>, error out=w221:errorcluster, "FP.State"=w218:T7)
                    n67 = case shown="Default" w218 {
                      tunnel: [w224 w227] -> w223
                      tunnel: w221 -> [w224 w226]
                      tunnel: w219 -> [_ w225]
                      frame "Invalid", "Closed" {
                      }
                      frame Default {
                        n68 = invoke class="VI" method="FP.Close"(reference=w225, error in=w226) -> (error out=w227:errorcluster)  [unwired: 1 in, 2 out]
                      }
                    }
                  }
                }
              }
              frame condition #1 {
              }
            }
            n69 = call <vilib>:"Add State(s) to Queue__jki_lib_state_machine.vi"("State(s) in (\"\")"=w201) -> ("States Out"=w200:string)  [unwired: 14 in]
          }
          frame "---------- Macro ----------" {
            # "Do not put any code in this frame.\n(It is a separator no-op. You can make a copy of this frame to create a new Macro frame)"
            n70 = call <vilib>:"Add State(s) to Queue__jki_lib_state_machine.vi"("State(s) in (\"\")"=w233) -> ("States Out"=w232:string)  [unwired: 14 in]
          }
          frame "Macro: Initialize" {
            # "Initialization Macro\n(This is called once, when the VI starts)"
            n71 = call <vilib>:"Add State(s) to Queue__jki_lib_state_machine.vi"("State(s) in Front (\"\")"="Data: Initialize\nInitialize Core Data\nEvents: Register", "State(s) in (\"\")"="Process: Sync", "State(s) at Back (\"\")"="UI: Initialize\nUI: Front Panel State >> Open") -> ("States Out"=w235:string)  [unwired: 12 in]
            n72 = call <vilib>:"Add State(s) to Queue__jki_lib_state_machine.vi"("State(s) in Front (\"\")"=w235, "State(s) in (\"\")"=w242) -> ("States Out"=w241:string)  [unwired: 13 in]
          }
          frame "Macro: Exit" {
            # "Exit Macro\n(This is called once, when the VI exits)"
            n73 = Unbundle By Name(w247) -> ("Core.Close Panel on Exit?"=w253:bool)
            n74 = Select(t="//UI: Front Panel State >> Close", s=w253, f="") -> (s? t:f=w250:string)
            n75 = call <vilib>:"Add State(s) to Queue__jki_lib_state_machine.vi"("State(s) in Front (\"\")"="Data: Cleanup\nEvents: Unregister", "State(s) in (\"\")"="Process: Sync", "State(s) at Back (\"\")"="Exit") -> ("States Out"=w244:string)  [unwired: 12 in]
            n76 = call <vilib>:"Add State(s) to Queue__jki_lib_state_machine.vi"("State(s) in (\"\")"=w250, "State(s) at Back (\"\")"=w244) -> ("States Out"=w249:string)  [unwired: 13 in]
            n77 = call <vilib>:"Add State(s) to Queue__jki_lib_state_machine.vi"("State(s) in Front (\"\")"=w249, "State(s) in (\"\")"=w256) -> ("States Out"=w255:string)  [unwired: 13 in]
          }
          frame "---------- Process ----------" {
            # "Template Separator\n(You can make a copy of, or modify, this frame)"
            n78 = call <vilib>:"Add State(s) to Queue__jki_lib_state_machine.vi"("State(s) in (\"\")"=w261) -> ("States Out"=w260:string)  [unwired: 14 in]
          }
          frame "Process: Sync" {
            n79 = Unbundle By Name(w269) -> ("Self Reference"=w265:refnum<class "SynchIO.USB4431.lvclass">)
            n80 = call <vilib>:"WaitOnProcessSync.vi"("error in (no error)"=w264, "SMO"=w265) -> ("error out"=w263:errorcluster, "Don't run?"=w268:bool)  [unwired: 7 in, 1 out]
            n81 = Select(t="Data: Cleanup\nEvents: Unregister\nExit", s=w268, f="") -> (s? t:f=w262:string)
            n82 = call <vilib>:"Add State(s) to Queue__jki_lib_state_machine.vi"("State(s) in Front (\"\")"=w262, "State(s) in (\"\")"=w272) -> ("States Out"=w271:string)  [unwired: 13 in]
          }
          frame "---------- Events ----------" {
            # "Template Separator\n(You can make a copy of, or modify, this frame)"
            n83 = call <vilib>:"Add State(s) to Queue__jki_lib_state_machine.vi"("State(s) in (\"\")"=w277) -> ("States Out"=w276:string)  [unwired: 14 in]
          }
          frame "Events: Register" {
            # "Expand to add\nmore events"
            # "Self Events (API Calls)"
            # "Base Class Protected Events"
            n84 = Unbundle By Name(w288) -> ("Self Reference"=w283:refnum<class "SynchIO.USB4431.lvclass">)
            n85 = call <vilib>:"GetProtectedEvents.vi"("SMO"=w283) -> ("error out"=w279:errorcluster, "SMO Protected Events"=w286:T10, "SMO out"=w285:refnum<class "SynchIO.USB4431.lvclass">)  [unwired: 8 in]
            n86 = call "SynchIO.USB4431.GetProtectedEvents.vi"("SynchIO.USB4431"=w285) -> ("error out"=w280:errorcluster, "Protected Events"=w284:T11)  [unwired: 8 in, 1 out]
            n87 = register-events(w286, w284) -> (reference out=w287:refnum<event-registration>, error out=w281:errorcluster)  [unwired: 2 in]
            n88 = Merge Errors(w282, w281, w280, w279) -> (w278:errorcluster)
            n89 = call <vilib>:"Add State(s) to Queue__jki_lib_state_machine.vi"("State(s) in (\"\")"=w290) -> ("States Out"=w289:string)  [unwired: 14 in]
          }
          frame "Events: Unregister" {
            n90 = Unregister For Events(event registration refnum=w293, error in=w292) -> (error out=w291:errorcluster)
            n91 = call <vilib>:"Clear Errors.vi"("error in (no error)"=w291) -> ()  [unwired: 5 in, 2 out]
            n92 = call <vilib>:"Add State(s) to Queue__jki_lib_state_machine.vi"("State(s) in (\"\")"=w296) -> ("States Out"=w295:string)  [unwired: 14 in]
          }
          frame "---------- API ----------" {
            n93 = call <vilib>:"Add State(s) to Queue__jki_lib_state_machine.vi"("State(s) in (\"\")"=w301) -> ("States Out"=w300:string)  [unwired: 14 in]
          }
          frame "API: NewData" {
            n94 = Unbundle By Name(w306) -> ("Self Reference"=w305:refnum<class "SynchIO.USB4431.lvclass">, "Your string data"=w302:string)
            n95 = call "SynchIO.USB4431.SetData.vi"("error in (no error)"=w304, "Data In"=w302, "SynchIO.USB4431"=w305) -> ("error out"=w303:errorcluster)  [unwired: 7 in, 1 out]
            n96 = call <vilib>:"Add State(s) to Queue__jki_lib_state_machine.vi"("State(s) in (\"\")"=w309, "State(s) at Back (\"\")"=w302) -> ("States Out"=w308:string)  [unwired: 13 in]
          }
          frame "API: Initialize" {
            n97 = call <vilib>:"Add State(s) to Queue__jki_lib_state_machine.vi"("State(s) in (\"\")"=w314) -> ("States Out"=w313:string)  [unwired: 14 in]
          }
          frame "----------USB-4431---------- " {
            n98 = call <vilib>:"Add State(s) to Queue__jki_lib_state_machine.vi"("State(s) in (\"\")"=w319) -> ("States Out"=w318:string)  [unwired: 14 in]
          }
          frame "USB-4431: Initialize" {
            w321 = 10123 items=["Finite Samples"=10178, "Continuous Samples"=10123] ("sample mode")
            n99 = Unbundle By Name(w328) -> ("AI Buffer Size (S)"=w320:i32, "AI Configuration"=w332:T2, "AO Configuration"=w331:T3, "Channels: AO"=w330:T4, "sampling info"=w329:cluster{"Fs":dbl, "#s":dbl})
            n100 = call "4431 USB - Create IO Channels.vi"("sample mode"=w321, "error in"=w325, "AI Buffer Size (S)"=w320, "sampling info"=w329, "AO"=w330, "AO Configuration"=w331, "AI Configuration"=w332) -> ("AO Task"=w322:refnum<k21>[], "AI task"=w323:refnum<k21>[], "error out"=w324:errorcluster)  [unwired: 1 in, 1 out]
            n101 = Bundle By Name(cluster=w328, "AI task"=w323, "AO Task"=w322) -> (w327:T8)
            n102 = call <vilib>:"Add State(s) to Queue__jki_lib_state_machine.vi"("State(s) in Front (\"\")"="USB-4431: ReadWrite" ("message"), "State(s) in (\"\")"=w335) -> ("States Out"=w334:string)  [unwired: 13 in]
          }
          frame "USB-4431: ReadWrite" {
            n103 = Unbundle By Name(w349) -> ("AI task"=w342:refnum<k21>[], "AO Task"=w343:refnum<k21>[], "sampling info"=w347:cluster{"Fs":dbl, "#s":dbl}, "AO Data"=w341:waveform(dbl)[], "Iteration"=w336:i32)
            n104 = Equal To 0?(x=w336) -> (x = 0?=w338:bool)
            n105 = call "4461 - AI AND AI - Read AND Write Uneven -- Array.vi"("Reset"=w338, "AO Array"=w341, "error in (no error)"=w339, "sampling info"=w347, "AO Task"=w343, "AI task"=w342) -> ("error out"=w344:errorcluster, "Input Signals"=w346:waveform(dbl)[])  [unwired: 4 in]
            "Signals Graph" <- w346
            n106 = Increment(x=w336) -> (x+1=w337:i32)
            n107 = case shown="True" "stop" {
              tunnel: ["USB-4431: ReadWrite" "USB-4431: Shutdown"] -> w345
              frame False {
              }
              frame True {
              }
            }
            n108 = Bundle By Name(cluster=w349, "AI Data"=w346, "Iteration"=w337) -> (w348:T8)
            n109 = call <vilib>:"Add State(s) to Queue__jki_lib_state_machine.vi"("State(s) in Front (\"\")"=w345, "State(s) in (\"\")"=w352) -> ("States Out"=w351:string)  [unwired: 13 in]
          }
          frame "USB-4431: Shutdown" {
            n110 = Unbundle By Name(w359) -> ("AI task"=w357:refnum<k21>[], "AO Task"=w356:refnum<k21>[])  [unwired: 5 out]
            n111 = Build Array (concatenate)(w357, w356) -> (w355:refnum<k21>[])
            n112 = for {
              tunnel: [w367] -> w361
              tunnel: w360 -> [w366]
              tunnel: w355 -> [w365] mode=indexing
              n113 = flat-sequence {
                tunnel: [w372] -> w368
                tunnel: w366 -> [w371]
                tunnel: w365 -> [w370]
                tunnel: [w373] -> w369
                tunnel: w368 -> [w373]
                tunnel: w369 -> [w376]
                tunnel: [w375] -> w367
                frame #0 {
                  n114 = call <vilib>:"DAQmx Stop Task.vi"("task/channels in"=w370, "error in"=w371) -> ("task out"=w372:refnum<k21>)  [unwired: 12 in, 1 out]
                }
                frame #1 {
                  n115 = Wait (ms)(milliseconds to wait=u32 50) -> ()  [unwired: 1 out]
                }
                frame #2 {
                  n116 = call <vilib>:"DAQmx Clear Task.vi"("task in"=w376) -> ("error out"=w375:errorcluster)  [unwired: 14 in]
                }
                frame #3 {
                  n117 = Wait (ms)(milliseconds to wait=u32 50) -> ()  [unwired: 1 out]
                }
              }
            }
            n118 = call <vilib>:"Add State(s) to Queue__jki_lib_state_machine.vi"("State(s) in Front (\"\")"="Macro: Exit", "State(s) in (\"\")"=w364) -> ("States Out"=w363:string)  [unwired: 13 in]
          }
        }
        n119 = call "StateHistory.vi"("Current State in"=w16) -> ("Current State out"=→"Current State":string, "delimited string"=→"State History":string)  [unwired: 9 in]
      }
    }
    frame Error {
    }
  }
  n120 = call-parent "Process.vi"("error in"=w7, "SynchIO"=w6) -> ("error out"=w4:errorcluster, "SynchIO out"=→"SynchIO.USB4431 out":refnum<class "SynchIO.USB4431.lvclass">)  [unwired: 8 in]
  n121 = Merge Errors(w4, w3) -> (→"error out":errorcluster)
